vi "Close SMU.vi"(8 "error in (no error)":errorcluster, 11 "IVI Refnum in":refnum<k15>) -> (0 "error out":errorcluster)   [LabVIEW 2018]
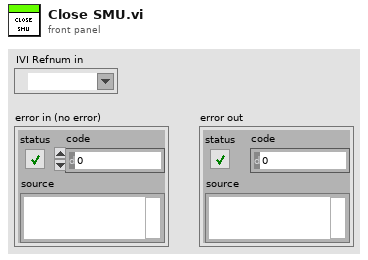
[diagram p1: front panel]
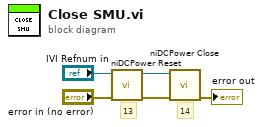
[diagram p0: block diagram]
diagram:
  # "14"
  # "13"
  n1 = call <instrlib>:"niDCPower Reset.vi"("error in (no error)"="error in (no error)", "instrument handle"="IVI Refnum in") -> ("error out"=w2:errorcluster, "instrument handle out"=w1:refnum<k15>)  [unwired: 2 in, 6 out]
  n2 = call <instrlib>:"niDCPower Close.vi"("error in (no error)"=w2, "instrument handle"=w1) -> ("error out"=→"error out":errorcluster)  [unwired: 9 out]
